vi "CONF digital RUN.vi"(8 "error in (no error)":errorcluster, 11 "Digital ref in":T1) -> (0 "error out":errorcluster, 3 "Digital ref out":T1)   [LabVIEW 2013]
doc: "Use this template to build a VI to use as a subVI."
uses:
  Kontrolki/KartaDAQ/CONF Digital Refnum.ctl
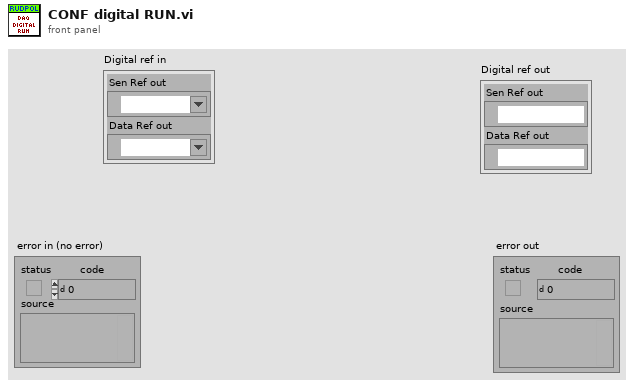
[diagram p1: front panel]
types:
  T1 = typedef "CONF Digital Refnum.ctl" = cluster{"Sen Ref out":refnum<k21>, "Data Ref out":refnum<k21>}
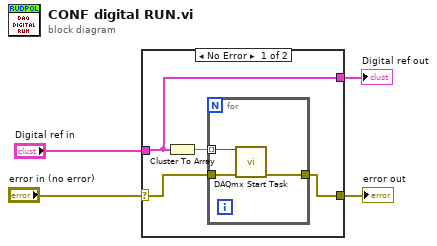
[diagram p0: block diagram]
diagram:
  n1 = case shown="No Error" "error in (no error)" {
    selector: "error in (no error)" -> [w6 w13]
    tunnel: [w5 w13] -> w3
    tunnel: "Digital ref in" -> [w7 w12]
    tunnel: [w7 w12] -> w1
    frame No Error {
      n2 = Cluster To Array(cluster=w7) -> (array=w8:refnum<k21>[])
      n3 = for {
        tunnel: w8 -> [w11] mode=indexing
        tunnel: w6 -> [w10]
        tunnel: [w9] -> w5
        n4 = call <vilib>:"DAQmx Start Task.vi"("task/channels in"=w11, "error in"=w10) -> ("error out"=w9:errorcluster)  [unwired: 12 in, 1 out]
      }
    }
    frame Error {
    }
  }
  "error out" <- w3
  "Digital ref out" <- w1
